vi "subVI_CONEX_setLimits.vi"(0 "CONEX Cluster":T1, 3 "Error IN":errorcluster, 4 "Retract Limit":dbl[](array[numeric]), 8 "Extend Limit":dbl[](array[numeric])) -> (6 "CONEX Cluster out":T1, 9 "error out":errorcluster)   [LabVIEW 2010]
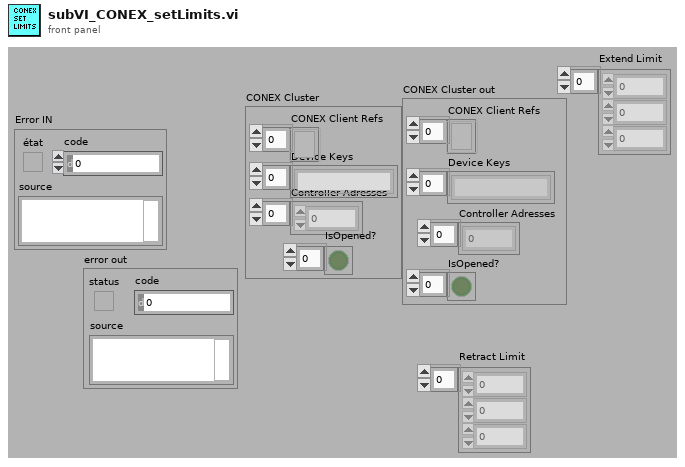
[diagram p1: front panel]
types:
  T1 = cluster{"CONEX Client Refs":refnum<k24>[], "Device Keys":string[], "Controller Adresses":i32[], "IsOpened?":bool[]}
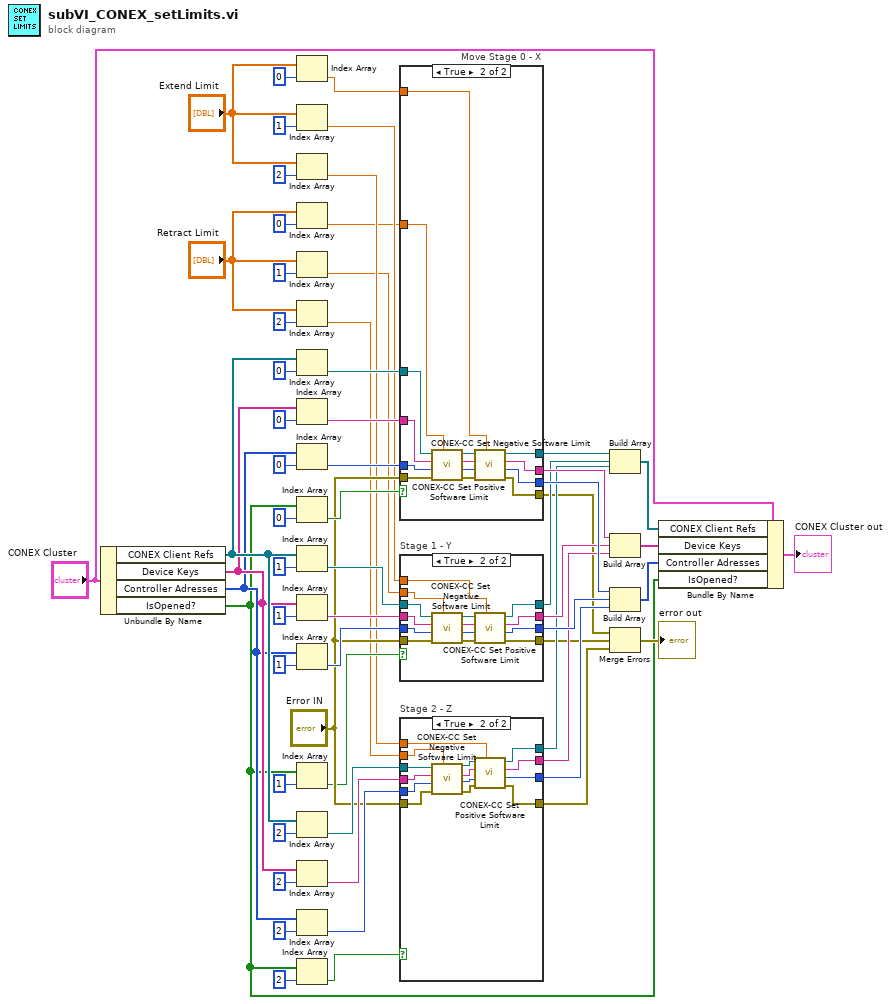
[diagram p0: block diagram]
diagram:
  n1 = Unbundle By Name("CONEX Cluster") -> ("CONEX Client Refs"=w58:refnum<k24>[], "Device Keys"=w53:string[], "Controller Adresses"=w48:i32[], "IsOpened?"=w17:bool[])
  n2 = Index Array(array="Extend Limit", index=0) -> (element=w7:dbl)
  n3 = Index Array(array="Extend Limit", index=1) -> (element=w9:dbl)
  n4 = Index Array(array="Extend Limit", index=2) -> (element=w11:dbl)
  n5 = Index Array(array="Retract Limit", index=0) -> (element=w8:dbl)
  n6 = Index Array(array="Retract Limit", index=1) -> (element=w10:dbl)
  n7 = Index Array(array="Retract Limit", index=2) -> (element=w12:dbl)
  n8 = Index Array(array=w58, index=0) -> (element=w57:refnum<k24>)
  n9 = Index Array(array=w53, index=0) -> (element=w52:string)
  n10 = Index Array(array=w48, index=0) -> (element=w47:i32)
  n11 = Index Array(array=w17, index=0) -> (element=w38:bool)
  n12 = Index Array(array=w58, index=1) -> (element=w36:refnum<k24>)
  n13 = Index Array(array=w53, index=1) -> (element=w34:string)
  n14 = Index Array(array=w48, index=1) -> (element=w31:i32)
  n15 = Index Array(array=w17, index=1) -> (element=w15:bool)
  n16 = Index Array(array=w58, index=2) -> (element=w35:refnum<k24>)
  n17 = Index Array(array=w53, index=2) -> (element=w33:string)
  n18 = Index Array(array=w48, index=2) -> (element=w32:i32)
  n19 = Index Array(array=w17, index=2) -> (element=w18:bool)
  n20 = case "Move Stage 0 - X" shown="True" w38 {
    tunnel: w57 -> [w62 w79]
    tunnel: w52 -> [w63 w78]
    tunnel: w47 -> [w64 w77]
    tunnel: "Error IN" -> [w65 w76]
    tunnel: [w62 w71] -> w46
    tunnel: [w63 w70] -> w45
    tunnel: [w64 w69] -> w44
    tunnel: [w65 w68] -> w20
    tunnel: w8 -> [_ w67]
    tunnel: w7 -> [_ w66]
    frame False {
    }
    frame True {
      n21 = call <userlib>:"CONEX-CC Set Negative Software Limit.vi"("Negative limit (left)"=w67, "Error IN"=w76, "Address IN"=w77, "deviceKey IN"=w78, "CONEX Client Ref IN"=w79) -> ("Error OUT"=w72:errorcluster, "Address OUT"=w73:i32, "deviceKey OUT"=w74:string, "CONEX Client Ref OUT"=w75:refnum<k24>)  [unwired: 1 in]
      n22 = call <userlib>:"CONEX-CC Set Positive Software Limit.vi"("Positive limit (right)"=w66, "Error IN"=w72, "Address IN"=w73, "deviceKey IN"=w74, "CONEX Client Ref IN"=w75) -> ("Error OUT"=w68:errorcluster, "Address OUT"=w69:i32, "deviceKey OUT"=w70:string, "CONEX Client Ref OUT"=w71:refnum<k24>)  [unwired: 1 in]
    }
  }
  n23 = case "Stage 1 - Y" shown="True" w15 {
    tunnel: w36 -> [w80 w97]
    tunnel: w34 -> [w81 w94]
    tunnel: w31 -> [w82 w96]
    tunnel: "Error IN" -> [w83 w95]
    tunnel: [w80 w89] -> w24
    tunnel: [w81 w88] -> w27
    tunnel: [w82 w87] -> w28
    tunnel: [w83 w86] -> w23
    tunnel: w10 -> [_ w85]
    tunnel: w9 -> [_ w84]
    frame False {
    }
    frame True {
      n24 = call <userlib>:"CONEX-CC Set Negative Software Limit.vi"("Negative limit (left)"=w85, "Error IN"=w95, "Address IN"=w96, "deviceKey IN"=w94, "CONEX Client Ref IN"=w97) -> ("Error OUT"=w90:errorcluster, "Address OUT"=w91:i32, "deviceKey OUT"=w92:string, "CONEX Client Ref OUT"=w93:refnum<k24>)  [unwired: 1 in]
      n25 = call <userlib>:"CONEX-CC Set Positive Software Limit.vi"("Positive limit (right)"=w84, "Error IN"=w90, "Address IN"=w91, "deviceKey IN"=w92, "CONEX Client Ref IN"=w93) -> ("Error OUT"=w86:errorcluster, "Address OUT"=w87:i32, "deviceKey OUT"=w88:string, "CONEX Client Ref OUT"=w89:refnum<k24>)  [unwired: 1 in]
    }
  }
  n26 = case "Stage 2 - Z" shown="True" w18 {
    tunnel: w35 -> [w98 w115]
    tunnel: w33 -> [w99 w114]
    tunnel: w32 -> [w100 w113]
    tunnel: "Error IN" -> [w101 w112]
    tunnel: [w98 w107] -> w25
    tunnel: [w99 w106] -> w26
    tunnel: [w100 w105] -> w29
    tunnel: [w101 w104] -> w22
    tunnel: w12 -> [_ w103]
    tunnel: w11 -> [_ w102]
    frame False {
    }
    frame True {
      n27 = call <userlib>:"CONEX-CC Set Negative Software Limit.vi"("Negative limit (left)"=w103, "Error IN"=w112, "Address IN"=w113, "deviceKey IN"=w114, "CONEX Client Ref IN"=w115) -> ("Error OUT"=w108:errorcluster, "Address OUT"=w109:i32, "deviceKey OUT"=w110:string, "CONEX Client Ref OUT"=w111:refnum<k24>)  [unwired: 1 in]
      n28 = call <userlib>:"CONEX-CC Set Positive Software Limit.vi"("Positive limit (right)"=w102, "Error IN"=w108, "Address IN"=w109, "deviceKey IN"=w110, "CONEX Client Ref IN"=w111) -> ("Error OUT"=w104:errorcluster, "Address OUT"=w105:i32, "deviceKey OUT"=w106:string, "CONEX Client Ref OUT"=w107:refnum<k24>)  [unwired: 1 in]
    }
  }
  n29 = Build Array(w46, w24, w25) -> (w43:refnum<k24>[])
  n30 = Build Array(w45, w27, w26) -> (w42:string[])
  n31 = Build Array(w44, w28, w29) -> (w41:i32[])
  n32 = Merge Errors(w20, w23, w22) -> (→"error out":errorcluster)
  n33 = Bundle By Name(cluster="CONEX Cluster", "CONEX Client Refs"=w43, "Device Keys"=w42, "Controller Adresses"=w41, "IsOpened?"=w17) -> (→"CONEX Cluster out":T1)
